vi "CheckMonthDateFolder.vi"(6 "file format (def: .tiff)":string=".tiff", 8 "Overwrite?":bool, 9 "Index":u32, 10 "File Name":string, 11 "Folder Path Control":path) -> (1 "Warning":bool, 2 "Message":string, 3 "File Path":path)   [LabVIEW 2014]
uses:
  <vilib>/regexp/Match Regular Expression.xnode
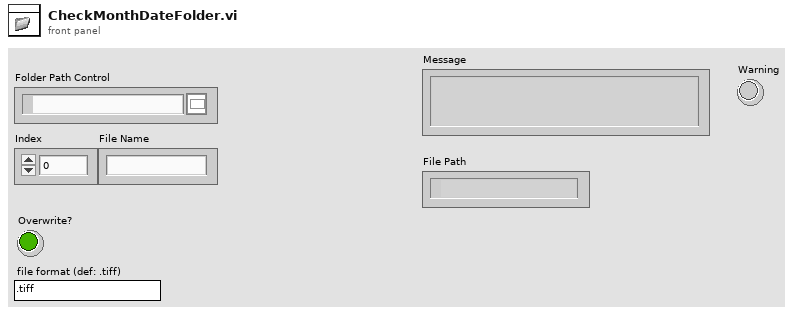
[diagram p1: front panel]
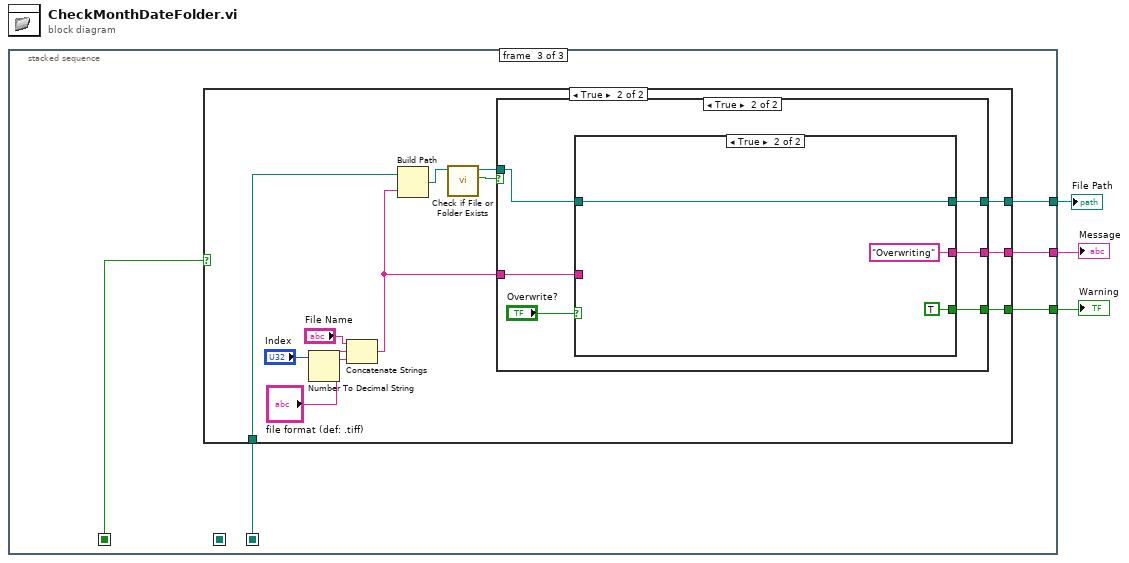
[diagram p0: block diagram]
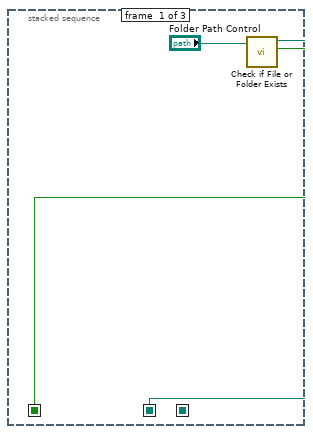
[diagram p2: hidden frame]
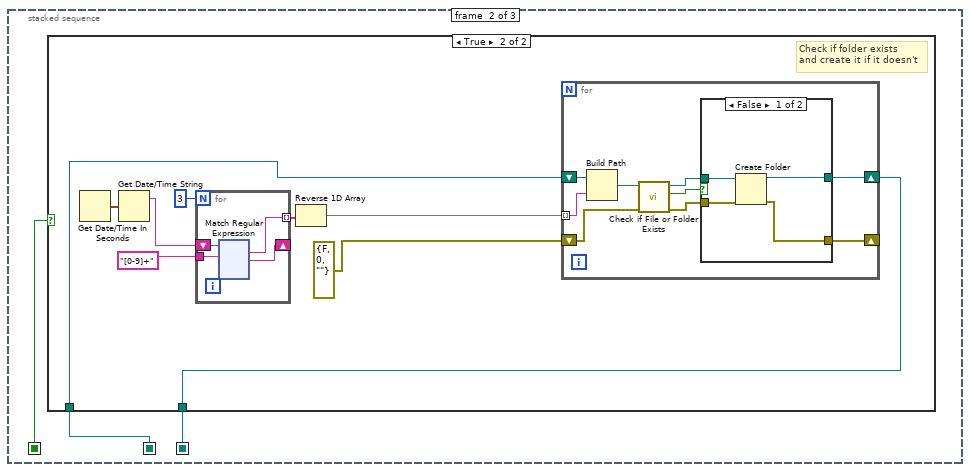
[diagram p3: hidden frame]
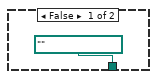
[diagram p4: hidden frame]
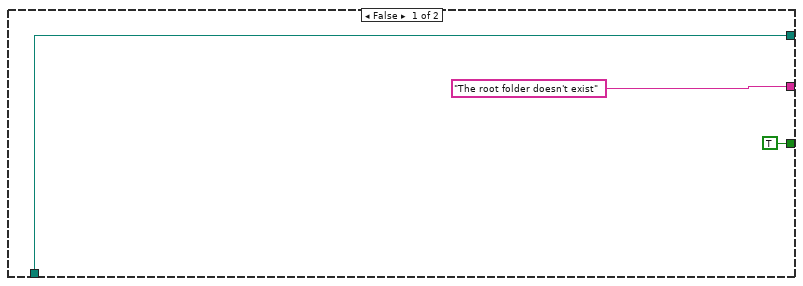
[diagram p6: hidden frame]
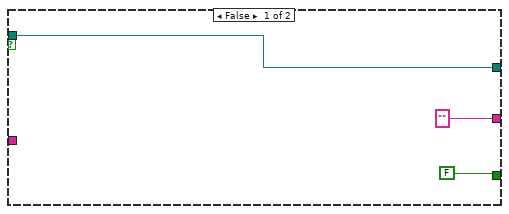
[diagram p7: hidden frame]
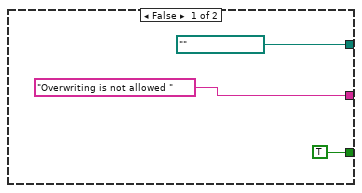
[diagram p8: hidden frame]
diagram:
  n1 = stacked-sequence {
    seq-local: [_ w9 _] -> [_ _ w157]
    seq-local: [w5 _ _] -> [_ w8 _]
    seq-local: [w4 _ _] -> [_ w7 w153]
    tunnel: [_ _ w156] -> w3
    tunnel: [_ _ w155] -> w2
    tunnel: [_ _ w154] -> w1
    frame #0 {
      n2 = call <vilib>:"Check if File or Folder Exists.vi"("path"="Folder Path Control") -> ("file or folder exists?"=w4:bool, "dup path"=w5:path)  [unwired: 8 in, 1 out]
    }
    frame #1 {
      n3 = case shown="True" w7 {
        tunnel: [path "" ("dup path") w12] -> w9
        tunnel: w8 -> [_ w11]
        frame False {
        }
        frame True {
          # "Check if folder exists\nand create it if it doesn't"
          n4 = Get Date/Time In Seconds() -> (seconds since 1Jan1904=w19:timestamp)
          n5 = Get Date/Time String(seconds (now)=w19) -> (date string=w18:string)  [unwired: 2 in, 1 out]
          n6 = for {
            N: 3 -> [_]
            tunnel: "[0-9]+" ("regular expression") -> [w37]
            tunnel: [w36] -> w15 mode=indexing
            shift-right: [w35] -> _
            shift-left: w18 -> [w38]
            n7 = xnode "Match Regular Expression"("input string"=w38, "regular expression"=w37) -> ("whole match"=w36:string, "after match"=w35:string)  [unwired: 4 in, 3 out]
          }
          n8 = Reverse 1D Array(array=w15) -> (reversed array=w14:string[])
          n9 = for {
            tunnel: w14 -> [w27] mode=indexing
            shift-right: [w21] -> w12
            shift-left: w11 -> [w28]
            shift-right: [w20] -> _
            shift-left: errorcluster {"status"=FALSE, "code"=0, "source"=""} ("error in (no error)") -> [w22]
            n10 = Build Path(base path=w28, name or relative path=w27) -> (appended path=w26:path)
            n11 = call <vilib>:"Check if File or Folder Exists.vi"("error in (no error)"=w22, "path"=w26) -> ("error out"=w23:errorcluster, "file or folder exists?"=w25:bool, "dup path"=w24:path)  [unwired: 7 in]
            n12 = case shown="False" w25 {
              tunnel: w24 -> [w32 w34]
              tunnel: w23 -> [w31 w33]
              tunnel: [w30 w34] -> w21
              tunnel: [w29 w33] -> w20
              frame False {
                n13 = Create Folder(path (use dialog)=w32, error in=w31) -> (created path=w30:path, error out=w29:errorcluster)  [unwired: 1 in, 1 out]
              }
              frame True {
              }
            }
          }
        }
      }
    }
    frame #2 {
      n14 = case shown="True" w153 {
        tunnel: w157 -> [w160 w169]
        tunnel: [w160 w167] -> w156
        tunnel: [TRUE w166] -> w155
        tunnel: ["The root folder doesn't exist" w163] -> w154
        frame False {
        }
        frame True {
          n15 = Number To Decimal String(number="Index") -> (decimal integer string=w170:string)  [unwired: 1 in]
          n16 = Concatenate Strings("File Name", w170, "file format (def: .tiff)") -> (w162:string)
          n17 = Build Path(base path=w169, name or relative path=w162) -> (appended path=w168:path)
          n18 = call <vilib>:"Check if File or Folder Exists.vi"("path"=w168) -> ("file or folder exists?"=w164:bool, "dup path"=w165:path)  [unwired: 8 in, 1 out]
          n19 = case shown="True" w164 {
            tunnel: [w175 w181] -> w167
            tunnel: [FALSE w180] -> w166
            tunnel: w165 -> [w175 w178]
            tunnel: ["" ("Message") w177] -> w163
            tunnel: w162 -> [_ w176]
            frame False {
            }
            frame True {
              n20 = case shown="True" "Overwrite?" {
                tunnel: [path "" ("File Path") w187] -> w181
                tunnel: [TRUE TRUE] -> w180
                tunnel: w178 -> [_ w187]
                tunnel: ["Overwriting is not allowed " ("Message") "Overwriting" ("Message")] -> w177
                tunnel: w176 -> [_ _]
                frame False {
                }
                frame True {
                }
              }
            }
          }
        }
      }
    }
  }
  "File Path" <- w3
  "Warning" <- w2
  "Message" <- w1
